vi "FTW-Endpoint-TCP-Bind-Captured.vi"(0 "FTW Endpoint":refnum<class "FTW-Endpoint-TCP.lvclass">, 5 "Connection":refnum<k5>, 11 "error in":errorcluster) -> (4 "FTW Endpoint out":refnum<class "FTW-Endpoint-TCP.lvclass">, 6 "Actual Endpoint Address":string, 8 "Actual Identity":string, 15 "error out":errorcluster)   [LabVIEW 2013, in "FTW-Endpoint-TCP.lvclass"]
uses:
  FTW-Endpoint-TCP.lvclass
  FTW-Endpoint-TCP.lvclass/FTW-Endpoint-TCP.ctl
panel:
  # "Inputs"
  # "Outputs"
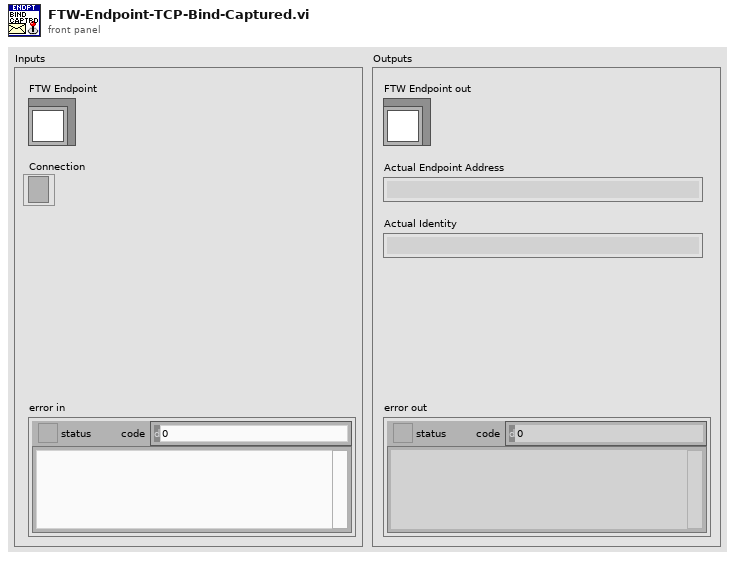
[diagram p1: front panel]
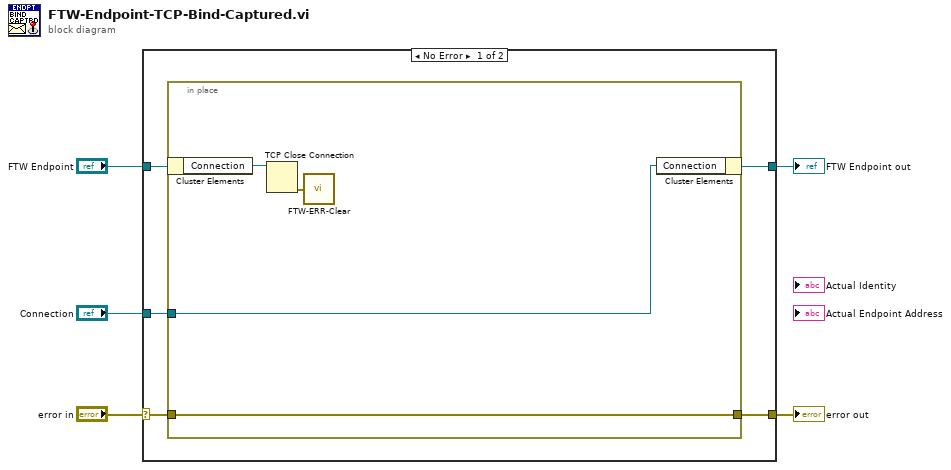
[diagram p0: block diagram]
diagram:
  n1 = case shown="No Error" "error in" {
    selector: "error in" -> [w9 w16]
    tunnel: [w6 w16] -> w5
    tunnel: [w7 w15] -> w3
    tunnel: "FTW Endpoint" -> [w10 w15]
    tunnel: "Connection" -> [w8 _]
    frame No Error {
      n2 = in-place {
        in-place-border: w9 -> [w12]
        in-place-border: [w12] -> w6
        in-place-border: w8 -> [w11]
        n3 = in-place-cluster #1(w10) -> ("Connection"=w14:refnum<k5>)
        n4 = TCP Close Connection(connection ID=w14) -> (error out=w13:errorcluster)  [unwired: 2 in, 1 out]
        n5 = call "FTW-ERR-Clear.vi"("error to snuff"=w13) -> ()  [unwired: 1 out]
        n6 = in-place-cluster #1("Connection"=w11) -> (w7:refnum<class "FTW-Endpoint-TCP.lvclass">)
      }
    }
    frame Error {
    }
  }
  "error out" <- w5
  "FTW Endpoint out" <- w3
